vi "SetAttribute.vi"(8 "error in (no error)":errorcluster, 9 "Value":variant, 10 "Name":string, 11 "reference in":refnum<class "MES_Local.lvclass">) -> (0 "error out":errorcluster, 3 "reference in":refnum<class "MES_Local.lvclass">)   [LabVIEW 2022 SP3, in "MES_Local.lvlib" / "MES_Local.lvclass"]
uses:
  MES_Local.lvclass
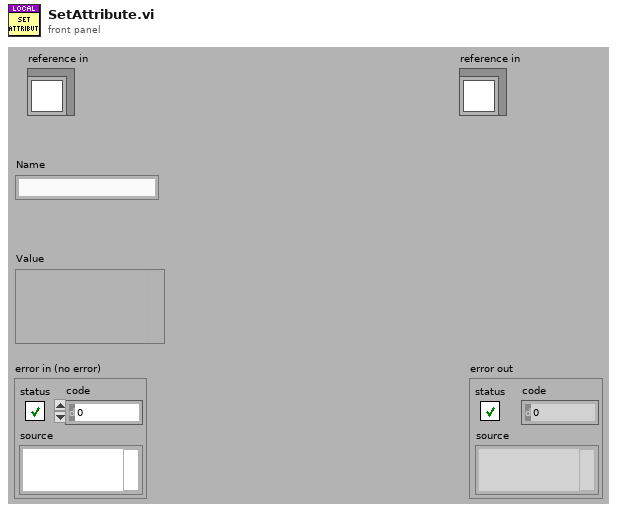
[diagram p1: front panel]
types:
  T1 = typedef "MES_Local.lvlib/MES_Local.lvclass/ObjectAttributes.ctl" = cluster{"Config":T2, "Logged_In?":bool, "AttributeNames":string[], "AttributeWritten":bool[], "ComponentNames":string[], "TestIndex":i32, "TestTag":string[], "Time Stamp":timestamp, "Employee":string, "Resource_Key":string, "Local Spec":path, "Login":refnum<class "Login_Base.lvclass">, "ReportPath":path, "Spec":T3, "StartTime":timestamp, "Role":string}
  T2 = typedef "MES_Local.lvlib/MES_Local.lvclass/Config.ctl" = cluster{"Results_Path":path}
  T3 = typedef "MES_Base.lvlibp/MES_Base.lvclass/Spec.ctl" = cluster{"Header":cluster{"Doctype":string, "Checksum":string, "DriverKey":string, "SpecId":string, "TransactionId":string, "AccountId":string, "SpecName":string, "WorkflowStep":string, "SerialNumber":string, "BatchNumber":string, "Status":enum16{"Pending", "Pass", "Fail"}, "Comment":string, "FirstFail":string, "Employee":string, "LocalMachine":string, "ResourceKey":string, "Date":string, "Time":string, "Duration":string, "DUT Position":i32}, "Components":cluster{"SerialNumber":string, "PartNumber":string, "Revision":string, "BatchNumber":string, "Name":string, "Description":string, "Attached":bool}[], "Attributes":cluster{"Name":string, "Description":string, "DataType":enum16{"NA", "String", "Boolean", "Int", "Dbl"}, "Value":variant, "DisplayFormat":string, "ReadOnly":bool, "Required":bool}[], "Tests":cluster{"Code":string, "Name":string, "Description":string, "Group":string, "IsGroup":bool, "Tag":string, "Method":string, "Parrameter":string, "DataType":enum16{"NA", "String", "Boolean", "Int", "Dbl"}, "Value":variant, "Status":enum16{"Pending", "Pass", "Fail"}, "LimitLo":variant, "LimitHi":variant, "StringMatch":string, "BooleanMatch":bool, "DisplayFormat":string, "Units":string, "TestTime":dbl}[]}
  T4 = cluster{"Name":string, "Description":string, "DataType":enum16{"NA", "String", "Boolean", "Int", "Dbl"}, "Value":variant, "DisplayFormat":string, "ReadOnly":bool, "Required":bool}[]
  T5 = cluster{"Name":string, "Description":string, "DataType":enum16{"NA", "String", "Boolean", "Int", "Dbl"}, "Value":variant, "DisplayFormat":string, "ReadOnly":bool, "Required":bool}
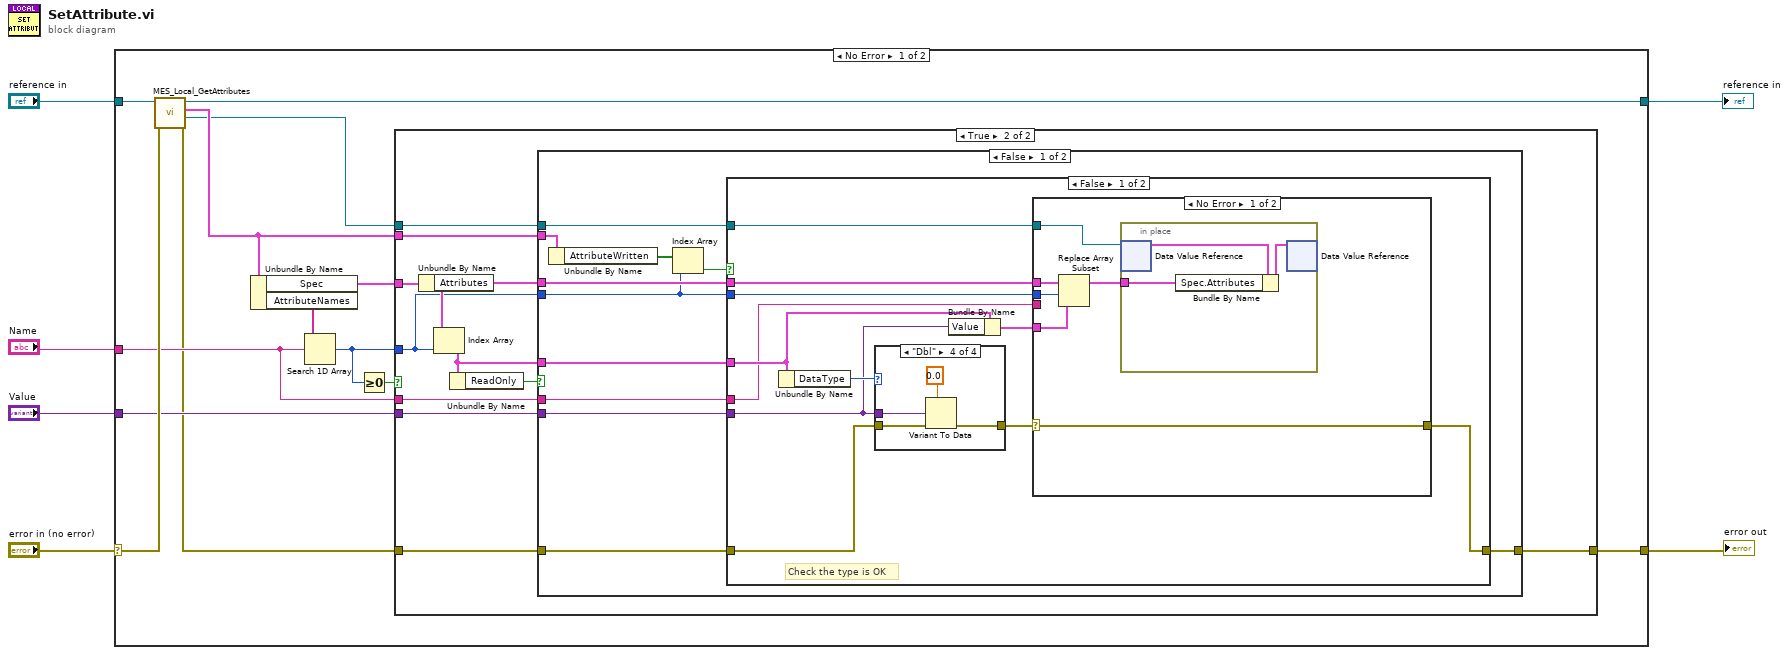
[diagram p0: block diagram]
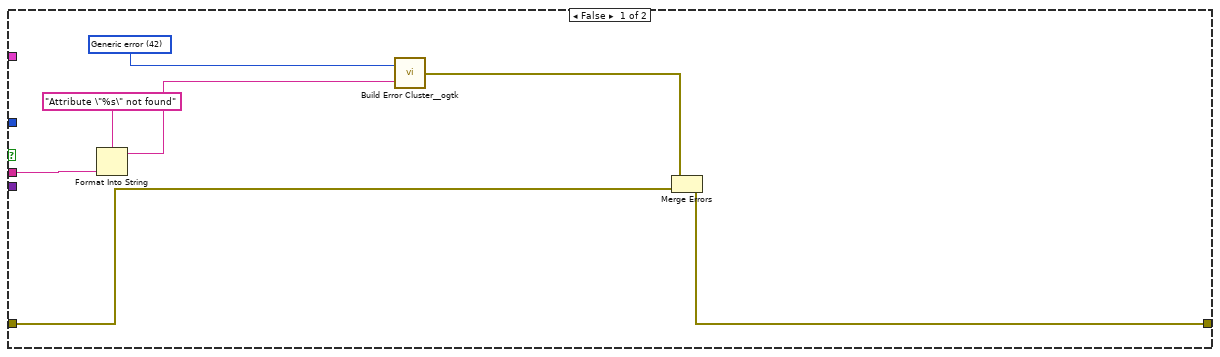
[diagram p2: hidden frame]
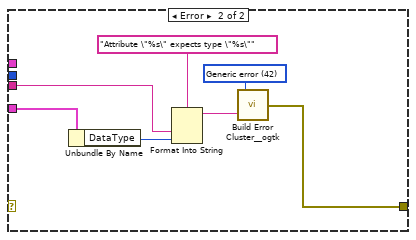
[diagram p3: hidden frame]
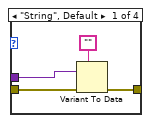
[diagram p4: hidden frame]
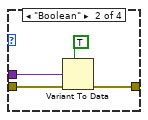
[diagram p5: hidden frame]
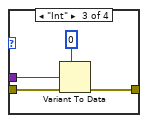
[diagram p6: hidden frame]
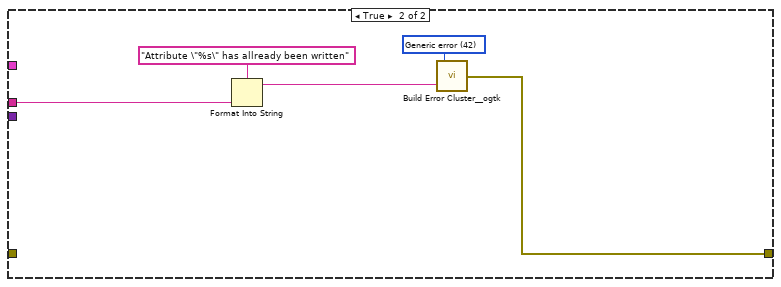
[diagram p7: hidden frame]
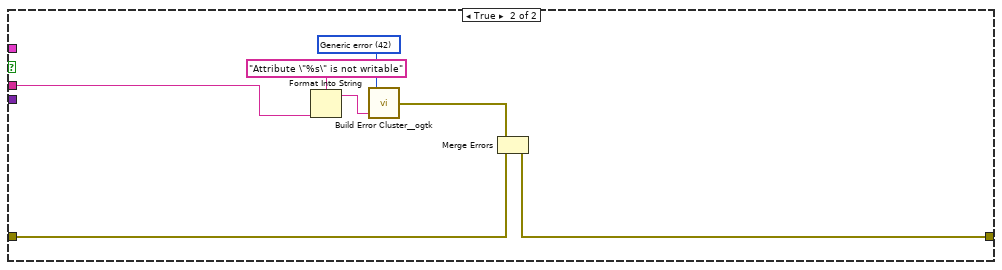
[diagram p8: hidden frame]
diagram:
  n1 = case shown="No Error" "error in (no error)" {
    selector: "error in (no error)" -> [w19 w105]
    tunnel: [w7 w105] -> w5
    tunnel: [w17 w104] -> w3
    tunnel: "reference in" -> [w18 w104]
    tunnel: "Name" -> [w10 _]
    tunnel: "Value" -> [w9 _]
    frame No Error {
      n2 = call "MES_Local_GetAttributes.vi"("error in (no error)"=w19, "reference in"=w18) -> ("error out"=w8:errorcluster, "DataRef"=w11:refnum<data-value>, "Data"=w12:T1, "reference out"=w17:refnum<class "MES_Local.lvclass">)  [unwired: 6 in]
      n3 = Unbundle By Name(w12) -> ("Spec"=w13:T3, "AttributeNames"=w16:string[])
      n4 = Search 1D Array(1D array=w16, element=w10) -> (index of element=w14:i32)  [unwired: 1 in]
      n5 = Greater Or Equal To 0?(x=w14) -> (x >= 0?=w15:bool)
      n6 = case shown="True" w15 {
        tunnel: w14 -> [_ w30]
        tunnel: w8 -> [w21 w35]
        tunnel: w10 -> [w25 w36]
        tunnel: [w20 w34] -> w7
        tunnel: w13 -> [_ w28]
        tunnel: w9 -> [_ w33]
        tunnel: w11 -> [_ w29]
        tunnel: w12 -> [_ w27]
        frame False {
          w26 = 42 items=["No error", "Argument error", "Memory is full", "Out of zone", "End of file", "File already open", "Generic file I/O error", "File not found", "File permission error", "Disk is full", "Duplicate path", "Too many files open", "System feature not enabled", "Resource file not found", "Cannot add resource", "Resource not found", "Image not found", "Image memory error", "Pen does not exist", "Config type invalid", "Config token not found", "Config parse error", "Config memory error", "Bad external code format", "Bad external code offset", "External code not present", "Null window", "Destroy window error", "Null menu", "Print aborted", "Bad print record", "Print driver error", "Windows error during printing", "Memory error during printing", "Print dialog error", "Generic print error", "Invalid device refnum", "Device not found", "Device parameter error", "Device unit error", "Cannot open device", "Device call aborted", "Generic error", "Cancelled by user", "Object ID too low", "Object ID too high", "Object not in heap", "Unknown heap", "Unknown object (invalid DefProc)", "Unknown object (DefProc not in table)", "Message out of range", "Invalid (null) method", "Unknown message", "Manager call not supported", "Bad address", "Network operation in progress", "Network operation timed out", "Connection is busy", "Network attribute not supported", "Network error", "Address in use", "System out of memory", "Connection aborted", "Connection refused", "Not connected", "Already connected", "Connection closed", "Initialization error (interapplication manager)", "Bad occurrence", "Wait on unbound occurrence handler", "Occurrence queue overflow", "Datalog type conflict", "Unused", "Unrecognized type (interapplication manager)", "Memory corrupt", "Failed to make temporary DLL", "Old CIN version", "Drag socket not found", "Failed to load drop-object", "Failed to register OLE object", "Failed to release OLE object", "Format specifier type mismatch", "Unknown format specifier", "Too few format specifiers", "Too many format specifiers", "Scan failed", "Newer CIN version", "Error converting to variant", "Runtime menu error", "Password tampered", "Variant attribute not found", "Incompatible variant data type", "Event data is not available", "Event Store is not present", "Occurrence is not found", "Event Queue is not created", "Event info is not available", "Refnum passed is NULL", "Error retrieving Class GUID", "Error retrieving CoClass GUID", "Error retrieving TypeLib GUID.", "Bad built application magic bytes.", "Specific driver is different from the specific driver associated with the Logical Name.", "There is no session opened to the class driver.", "Max Error", "MAX - Error with config objects", "MAX - Error loading configuration", "MAX - Group not supported"]
          n7 = Format Into String(format string="Attribute \"%s\" not found", w25) -> (resulting string=w23:string)  [unwired: 2 in, 1 out]
          n8 = call <userlib>:"Build Error Cluster__ogtk.vi"("String to Prepend to source (\"\")"=w23, "code"=w26) -> ("error out"=w22:errorcluster)
          n9 = Merge Errors(w22, w21) -> (w20:errorcluster)
        }
        frame True {
          n10 = Unbundle By Name(w28) -> ("Attributes"=w31:T4)
          n11 = Index Array(array=w31, index=w30) -> (element=w32:T5)
          n12 = Unbundle By Name(w32) -> ("ReadOnly"=w37:bool)
          n13 = case shown="False" w37 {
            tunnel: w35 -> [w48 w98]
            tunnel: w36 -> [w38 w101]
            tunnel: [w46 w97] -> w34
            tunnel: w33 -> [w47 _]
            tunnel: w32 -> [w43 _]
            tunnel: w31 -> [w45 _]
            tunnel: w30 -> [w40 _]
            tunnel: w29 -> [w44 _]
            tunnel: w27 -> [w42 _]
            frame False {
              n14 = Unbundle By Name(w42) -> ("AttributeWritten"=w41:bool[])
              n15 = Index Array(array=w41, index=w40) -> (element=w39:bool)
              n16 = case shown="False" w39 {
                tunnel: w48 -> [w58 _]
                tunnel: w47 -> [w57 _]
                tunnel: [w49 w92] -> w46
                tunnel: w45 -> [w55 _]
                tunnel: w44 -> [w52 _]
                tunnel: w43 -> [w54 _]
                tunnel: w40 -> [w53 _]
                tunnel: w38 -> [w50 w95]
                frame False {
                  # "Check the type is OK"
                  n17 = Unbundle By Name(w54) -> ("DataType"=w59:enum16{"NA", "String", "Boolean", "Int", "Dbl"})
                  n18 = case shown="\"Dbl\"" w59 {
                    tunnel: w57 -> [w78 w82 w87 w91]
                    tunnel: w58 -> [w79 w81 w86 w90]
                    tunnel: [w77 w80 w85 w89] -> w51
                    frame "String", Default {
                      n19 = Variant To Data(error in=w79, type="", Variant=w78) -> (error out=w77:errorcluster)  [unwired: 1 out]
                    }
                    frame "Boolean" {
                      n20 = Variant To Data(error in=w81, type=TRUE, Variant=w82) -> (error out=w80:errorcluster)  [unwired: 1 out]
                    }
                    frame "Int" {
                      n21 = Variant To Data(error in=w86, type=0, Variant=w87) -> (error out=w85:errorcluster)  [unwired: 1 out]
                    }
                    frame "Dbl" {
                      n22 = Variant To Data(error in=w90, type=0.0, Variant=w91) -> (error out=w89:errorcluster)  [unwired: 1 out]
                    }
                  }
                  n23 = Bundle By Name(cluster=w54, "Value"=w57) -> (w56:T5)
                  n24 = case shown="No Error" w51 {
                    selector: w51 -> [w60 _]
                    tunnel: w56 -> [w64 w73]
                    tunnel: w55 -> [w65 _]
                    tunnel: w53 -> [w63 _]
                    tunnel: w52 -> [w62 _]
                    tunnel: w50 -> [_ w70]
                    tunnel: [w60 w69] -> w49
                    frame No Error {
                      n25 = Replace Array Subset(array=w65, new element=w64, index=w63) -> (w61:T4)
                      n26 = in-place {
                        in-place-border: w61 -> [w66]
                        n27 = in-place-dvr #1(w62) -> (w68:T1)  [unwired: 1 out]
                        n28 = Bundle By Name(cluster=w68, "Spec.Attributes"=w66) -> (w67:T1)
                        n29 = in-place-dvr #1(w67) -> ()  [unwired: 2 out]
                      }
                    }
                    frame Error {
                      w75 = 42 items=["No error", "Argument error", "Memory is full", "Out of zone", "End of file", "File already open", "Generic file I/O error", "File not found", "File permission error", "Disk is full", "Duplicate path", "Too many files open", "System feature not enabled", "Resource file not found", "Cannot add resource", "Resource not found", "Image not found", "Image memory error", "Pen does not exist", "Config type invalid", "Config token not found", "Config parse error", "Config memory error", "Bad external code format", "Bad external code offset", "External code not present", "Null window", "Destroy window error", "Null menu", "Print aborted", "Bad print record", "Print driver error", "Windows error during printing", "Memory error during printing", "Print dialog error", "Generic print error", "Invalid device refnum", "Device not found", "Device parameter error", "Device unit error", "Cannot open device", "Device call aborted", "Generic error", "Cancelled by user", "Object ID too low", "Object ID too high", "Object not in heap", "Unknown heap", "Unknown object (invalid DefProc)", "Unknown object (DefProc not in table)", "Message out of range", "Invalid (null) method", "Unknown message", "Manager call not supported", "Bad address", "Network operation in progress", "Network operation timed out", "Connection is busy", "Network attribute not supported", "Network error", "Address in use", "System out of memory", "Connection aborted", "Connection refused", "Not connected", "Already connected", "Connection closed", "Initialization error (interapplication manager)", "Bad occurrence", "Wait on unbound occurrence handler", "Occurrence queue overflow", "Datalog type conflict", "Unused", "Unrecognized type (interapplication manager)", "Memory corrupt", "Failed to make temporary DLL", "Old CIN version", "Drag socket not found", "Failed to load drop-object", "Failed to register OLE object", "Failed to release OLE object", "Format specifier type mismatch", "Unknown format specifier", "Too few format specifiers", "Too many format specifiers", "Scan failed", "Newer CIN version", "Error converting to variant", "Runtime menu error", "Password tampered", "Variant attribute not found", "Incompatible variant data type", "Event data is not available", "Event Store is not present", "Occurrence is not found", "Event Queue is not created", "Event info is not available", "Refnum passed is NULL", "Error retrieving Class GUID", "Error retrieving CoClass GUID", "Error retrieving TypeLib GUID.", "Bad built application magic bytes.", "Specific driver is different from the specific driver associated with the Logical Name.", "There is no session opened to the class driver.", "Max Error", "MAX - Error with config objects", "MAX - Error loading configuration", "MAX - Group not supported"]
                      n30 = Unbundle By Name(w73) -> ("DataType"=w72:enum16{"NA", "String", "Boolean", "Int", "Dbl"})
                      n31 = Format Into String(format string="Attribute \"%s\" expects type \"%s\"", w70, w72) -> (resulting string=w74:string)  [unwired: 2 in, 1 out]
                      n32 = call <userlib>:"Build Error Cluster__ogtk.vi"("String to Prepend to source (\"\")"=w74, "code"=w75) -> ("error out"=w69:errorcluster)
                    }
                  }
                }
                frame True {
                  w94 = 42 items=["No error", "Argument error", "Memory is full", "Out of zone", "End of file", "File already open", "Generic file I/O error", "File not found", "File permission error", "Disk is full", "Duplicate path", "Too many files open", "System feature not enabled", "Resource file not found", "Cannot add resource", "Resource not found", "Image not found", "Image memory error", "Pen does not exist", "Config type invalid", "Config token not found", "Config parse error", "Config memory error", "Bad external code format", "Bad external code offset", "External code not present", "Null window", "Destroy window error", "Null menu", "Print aborted", "Bad print record", "Print driver error", "Windows error during printing", "Memory error during printing", "Print dialog error", "Generic print error", "Invalid device refnum", "Device not found", "Device parameter error", "Device unit error", "Cannot open device", "Device call aborted", "Generic error", "Cancelled by user", "Object ID too low", "Object ID too high", "Object not in heap", "Unknown heap", "Unknown object (invalid DefProc)", "Unknown object (DefProc not in table)", "Message out of range", "Invalid (null) method", "Unknown message", "Manager call not supported", "Bad address", "Network operation in progress", "Network operation timed out", "Connection is busy", "Network attribute not supported", "Network error", "Address in use", "System out of memory", "Connection aborted", "Connection refused", "Not connected", "Already connected", "Connection closed", "Initialization error (interapplication manager)", "Bad occurrence", "Wait on unbound occurrence handler", "Occurrence queue overflow", "Datalog type conflict", "Unused", "Unrecognized type (interapplication manager)", "Memory corrupt", "Failed to make temporary DLL", "Old CIN version", "Drag socket not found", "Failed to load drop-object", "Failed to register OLE object", "Failed to release OLE object", "Format specifier type mismatch", "Unknown format specifier", "Too few format specifiers", "Too many format specifiers", "Scan failed", "Newer CIN version", "Error converting to variant", "Runtime menu error", "Password tampered", "Variant attribute not found", "Incompatible variant data type", "Event data is not available", "Event Store is not present", "Occurrence is not found", "Event Queue is not created", "Event info is not available", "Refnum passed is NULL", "Error retrieving Class GUID", "Error retrieving CoClass GUID", "Error retrieving TypeLib GUID.", "Bad built application magic bytes.", "Specific driver is different from the specific driver associated with the Logical Name.", "There is no session opened to the class driver.", "Max Error", "MAX - Error with config objects", "MAX - Error loading configuration", "MAX - Group not supported"]
                  n33 = Format Into String(format string="Attribute \"%s\" has allready been written", w95) -> (resulting string=w93:string)  [unwired: 2 in, 1 out]
                  n34 = call <userlib>:"Build Error Cluster__ogtk.vi"("String to Prepend to source (\"\")"=w93, "code"=w94) -> ("error out"=w92:errorcluster)
                }
              }
            }
            frame True {
              w103 = 42 items=["No error", "Argument error", "Memory is full", "Out of zone", "End of file", "File already open", "Generic file I/O error", "File not found", "File permission error", "Disk is full", "Duplicate path", "Too many files open", "System feature not enabled", "Resource file not found", "Cannot add resource", "Resource not found", "Image not found", "Image memory error", "Pen does not exist", "Config type invalid", "Config token not found", "Config parse error", "Config memory error", "Bad external code format", "Bad external code offset", "External code not present", "Null window", "Destroy window error", "Null menu", "Print aborted", "Bad print record", "Print driver error", "Windows error during printing", "Memory error during printing", "Print dialog error", "Generic print error", "Invalid device refnum", "Device not found", "Device parameter error", "Device unit error", "Cannot open device", "Device call aborted", "Generic error", "Cancelled by user", "Object ID too low", "Object ID too high", "Object not in heap", "Unknown heap", "Unknown object (invalid DefProc)", "Unknown object (DefProc not in table)", "Message out of range", "Invalid (null) method", "Unknown message", "Manager call not supported", "Bad address", "Network operation in progress", "Network operation timed out", "Connection is busy", "Network attribute not supported", "Network error", "Address in use", "System out of memory", "Connection aborted", "Connection refused", "Not connected", "Already connected", "Connection closed", "Initialization error (interapplication manager)", "Bad occurrence", "Wait on unbound occurrence handler", "Occurrence queue overflow", "Datalog type conflict", "Unused", "Unrecognized type (interapplication manager)", "Memory corrupt", "Failed to make temporary DLL", "Old CIN version", "Drag socket not found", "Failed to load drop-object", "Failed to register OLE object", "Failed to release OLE object", "Format specifier type mismatch", "Unknown format specifier", "Too few format specifiers", "Too many format specifiers", "Scan failed", "Newer CIN version", "Error converting to variant", "Runtime menu error", "Password tampered", "Variant attribute not found", "Incompatible variant data type", "Event data is not available", "Event Store is not present", "Occurrence is not found", "Event Queue is not created", "Event info is not available", "Refnum passed is NULL", "Error retrieving Class GUID", "Error retrieving CoClass GUID", "Error retrieving TypeLib GUID.", "Bad built application magic bytes.", "Specific driver is different from the specific driver associated with the Logical Name.", "There is no session opened to the class driver.", "Max Error", "MAX - Error with config objects", "MAX - Error loading configuration", "MAX - Group not supported"]
              n35 = Format Into String(format string="Attribute \"%s\" is not writable", w101) -> (resulting string=w100:string)  [unwired: 2 in, 1 out]
              n36 = call <userlib>:"Build Error Cluster__ogtk.vi"("String to Prepend to source (\"\")"=w100, "code"=w103) -> ("error out"=w99:errorcluster)
              n37 = Merge Errors(w99, w98) -> (w97:errorcluster)
            }
          }
        }
      }
    }
    frame Error {
    }
  }
  "error out" <- w5
  "reference in" <- w3
